vi "Caller.vi"(0 "Multiply in":refnum<class "Multiply.lvclass">, 2 "DVR In":refnum<data-value>, 11 "Error In":errorcluster) -> (4 "Multiply out":refnum<class "Multiply.lvclass">, 15 "Error Out":errorcluster)   [LabVIEW 2023, in "Multiply.lvclass"]
doc: "The VI opens the reference of operation UI that allows user to perform multiplication operation and runs the VI in the background."
uses:
  Multiply.lvclass
  Arithemtic Operation/Arithemetic Operation.lvclass
  Multiply.lvclass/Multiply.ctl
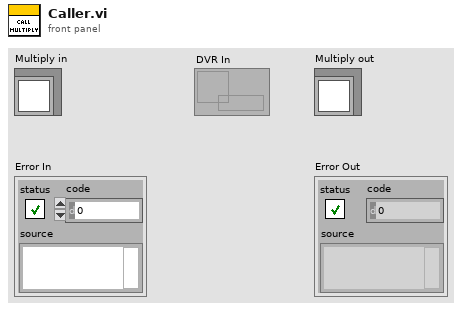
[diagram p1: front panel]
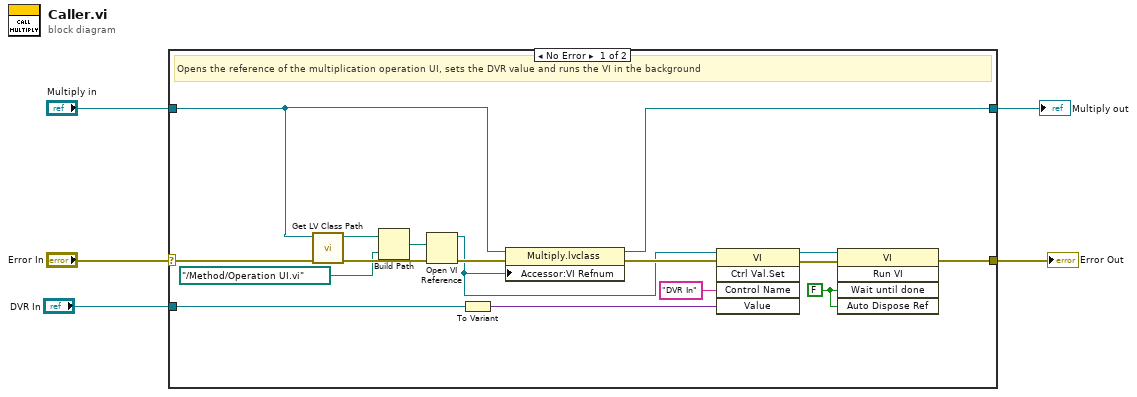
[diagram p0: block diagram]
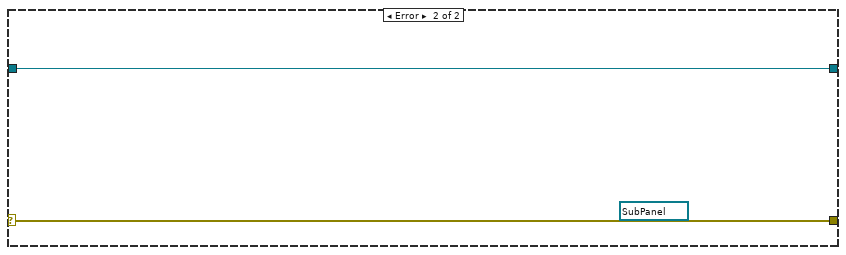
[diagram p2: hidden frame]
diagram:
  n1 = case shown="No Error" "Error In" {
    selector: "Error In" -> [w18 w24]
    tunnel: [w6 w24] -> w4
    tunnel: [w17 w23] -> w2
    tunnel: "Multiply in" -> [w16 w23]
    tunnel: "DVR In" -> [w8 _]
    frame No Error {
      w11 = FALSE ("Wait Until Done")
      # "Opens the reference of the multiplication operation UI, sets the DVR value and runs the VI in the background"
      n2 = call <vilib>:"Get LV Class Path.vi"("error in (no error)"=w18, "object"=w16) -> ("error out"=w22:errorcluster, "class path"=w21:path)  [unwired: 8 in]
      n3 = Build Path(base path=w21, name or relative path=path "../Method/Operation UI.vi") -> (appended path=w19:path)
      n4 = Open VI Reference(vi path=w19, error in (no error)=w22) -> (vi reference=w9:refnum<vi>, error out=w15:errorcluster)  [unwired: 4 in]
      n5 = To Variant(anything=w8) -> (Variant=w7:variant)
      n6 = property class="Multiply.lvclass"(reference=w16, error in=w15, "Accessor:VI Refnum"=w9) -> (reference out=w17:refnum<class "Multiply.lvclass">, error out=w10:errorcluster)
      n7 = invoke class="VI" method="Ctrl Val.Set"(reference=w9, error in=w10, "Control Name"="DVR In", "Value"=w7) -> (reference out=w13:refnum<vi>, error out=w12:errorcluster)  [unwired: 1 in, 3 out]
      n8 = invoke class="VI" method="Run VI"(reference=w13, error in=w12, "Wait until done"=w11, "Auto Dispose Ref"=w11) -> (error out=w6:errorcluster)  [unwired: 1 in, 4 out]
    }
    frame Error {
      (unwired) refnum<vi> refnum ("Sub Panel")
    }
  }
  "Error Out" <- w4
  "Multiply out" <- w2
